vi "Init Device.vi"(7 "Layout Ref":refnum<vi>, 8 "error in (no error)":errorcluster, 10 "Chan# Array":i32[](array[numeric]), 11 "SRS_DS345 in":refnum<class "SRS_DS345.lvclass">) -> (0 "error out":errorcluster, 3 "SRS_DS345 out":refnum<class "SRS_DS345.lvclass">)   [LabVIEW 2013, in "SRS_DS345.lvclass"]
doc: "Initialize the correct columns and their default appearance.\nUse the front panel to change default appearance of the device in the Add/Manage devices.\n\nOpen a specific device implementation for details."
uses:
  SRS_DS345.lvclass
  TypeDefs/ColumnAppearCluster.ctl
  ColumnVIs/SingleValCol/SingleValCol.lvclass
  ColumnVIs/SingleValMenuCol/SingleValMenuCol.lvclass
  ColumnVIs/Column/Column.lvclass
panel:
  in  "MenuItemList":string[](array[string])=["Sine", "Square", "Triangle", "Ramp"]
  in  "Function Type Column Defaults":T1={"Column Name"="Func Type", "Width"=30, "Bkgd"=[16448250], "Text"=[0]}
  in  "Offset Column Defaults":T1={"Column Name"="Offset", "Width"=30, "Bkgd"=[16448250], "Text"=[0]}
  in  "Amplitude Column Defaults":T1={"Column Name"="Amplitude", "Width"=30, "Bkgd"=[16448250], "Text"=[0]}
  in  "Freq Column Defaults":T1={"Column Name"="Frequency", "Width"=30, "Bkgd"=[16448250], "Text"=[0]}
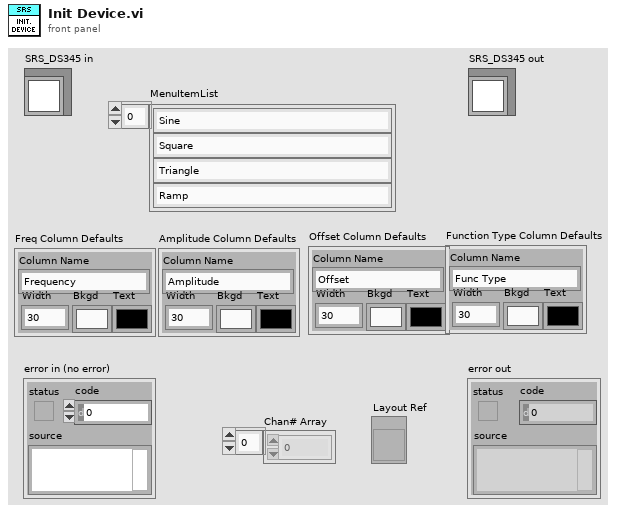
[diagram p1: front panel]
types:
  T1 = typedef "ColumnAppearCluster.ctl" = cluster{"Column Name":string, "Width":u32, "Bkgd":u32[], "Text":u32[]}
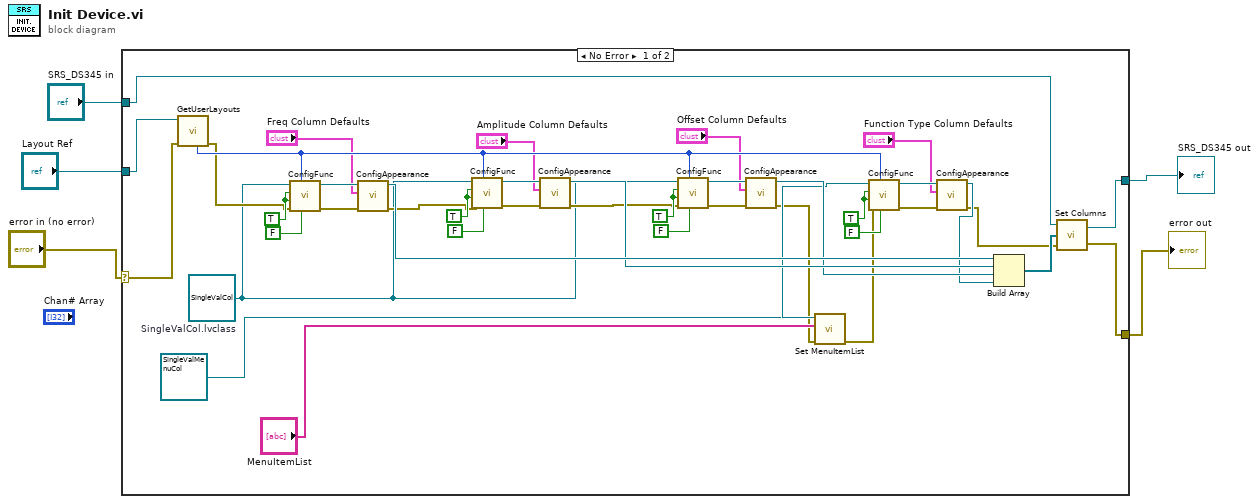
[diagram p0: block diagram]
diagram:
  n1 = case shown="No Error" "error in (no error)" {
    selector: "error in (no error)" -> [w45 w47]
    tunnel: "SRS_DS345 in" -> [w26 w48]
    tunnel: [w25 w48] -> w3
    tunnel: [w16 w47] -> w2
    tunnel: "Layout Ref" -> [w46 _]
    frame No Error {
      w37 = TRUE ("Disableable? (True)")
      w39 = TRUE ("Disableable? (True)")
      w41 = TRUE ("Disableable? (True)")
      w43 = TRUE ("Disableable? (True)")
      w11 = refnum<class "SingleValCol.lvclass"> refnum  # SingleValCol.lvclass
      n2 = call "GetUserLayouts.vi"("error in (no error)"=w45, "Layout Ring Refnum"=w46) -> ("error out"=w24:errorcluster, "Num User Layouts"=w36:i32)  [unwired: 5 in, 3 out]
      n3 = call "ConfigFunc.vi"("isRampable? (True"=FALSE, "Num Layouts (ignored)"=w36, "error in (no error)"=w24, "isVariable? (True)"=w43, "Disableable? (True)"=w43, "Column in"=w11) -> ("error out"=w23:errorcluster, "Column out"=w44:refnum<class "SingleValCol.lvclass">)  [unwired: 4 in]
      n4 = call "ConfigAppearance.vi"("error in (no error)"=w23, "Column Appearance"="Freq Column Defaults", "Column in"=w44) -> ("error out"=w22:errorcluster, "Column out"=w31:refnum<class "SingleValCol.lvclass">)  [unwired: 7 in]
      n5 = call "ConfigFunc.vi"("isRampable? (True"=FALSE, "Num Layouts (ignored)"=w36, "error in (no error)"=w22, "isVariable? (True)"=w41, "Disableable? (True)"=w41, "Column in"=w11) -> ("error out"=w21:errorcluster, "Column out"=w42:refnum<class "SingleValCol.lvclass">)  [unwired: 4 in]
      n6 = call "ConfigAppearance.vi"("error in (no error)"=w21, "Column Appearance"="Amplitude Column Defaults", "Column in"=w42) -> ("error out"=w20:errorcluster, "Column out"=w30:refnum<class "SingleValCol.lvclass">)  [unwired: 7 in]
      n7 = call "ConfigFunc.vi"("isRampable? (True"=FALSE, "Num Layouts (ignored)"=w36, "error in (no error)"=w20, "isVariable? (True)"=w39, "Disableable? (True)"=w39, "Column in"=w11) -> ("error out"=w19:errorcluster, "Column out"=w40:refnum<class "SingleValCol.lvclass">)  [unwired: 4 in]
      n8 = call "ConfigAppearance.vi"("error in (no error)"=w19, "Column Appearance"="Offset Column Defaults", "Column in"=w40) -> ("error out"=w8:errorcluster, "Column out"=w29:refnum<class "SingleValCol.lvclass">)  [unwired: 7 in]
      n9 = call-dynamic "Set MenuItemList.vi"("error in (no error)"=w8, "MenuItemList"="MenuItemList", "MenuCol in"=refnum<class "SingleValMenuCol.lvclass"> refnum ("SingleValMenuCol.lvclass")) -> ("error out"=w7:errorcluster, "MenuCol out"=w10:refnum<class "SingleValMenuCol.lvclass">)  [unwired: 7 in]
      n10 = call "ConfigFunc.vi"("isRampable? (True"=FALSE, "Num Layouts (ignored)"=w36, "error in (no error)"=w7, "isVariable? (True)"=w37, "Disableable? (True)"=w37, "Column in"=w10) -> ("error out"=w18:errorcluster, "Column out"=w38:refnum<class "SingleValMenuCol.lvclass">)  [unwired: 4 in]
      n11 = call "ConfigAppearance.vi"("error in (no error)"=w18, "Column Appearance"="Function Type Column Defaults", "Column in"=w38) -> ("error out"=w17:errorcluster, "Column out"=w28:refnum<class "SingleValMenuCol.lvclass">)  [unwired: 7 in]
      n12 = Build Array(w31, w30, w29, w28) -> (w27:refnum<class "Column.lvclass">[])
      n13 = call-dynamic "Set Columns.vi"("error in (no error)"=w17, "Columns"=w27, "Device in"=w26) -> ("error out"=w16:errorcluster, "Device out"=w25:refnum<class "SRS_DS345.lvclass">)  [unwired: 1 in]
    }
    frame Error {
    }
  }
  "error out" <- w2
  "SRS_DS345 out" <- w3
